vi "Cleanup.vi"(8 "error in (no error)":errorcluster, 11 "DC Brick in":refnum<class "DC Brick.lvclass">) -> (0 "error out":errorcluster)   [LabVIEW 2011, in "Tinkerforge.lvlib" / "DC Brick.lvclass"]
doc: "This VI is the child implementation of \"Cleanup.vi\" and releases all synchronization objects of this child object."
uses:
  DC Brick.lvclass
  DC Brick.lvclass/DC Brick.ctl
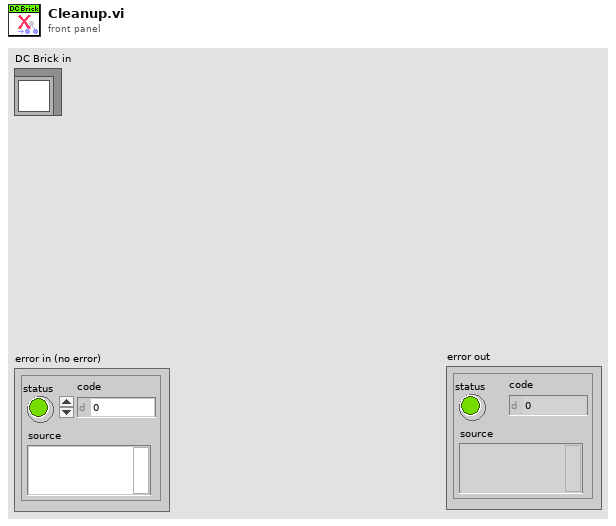
[diagram p1: front panel]
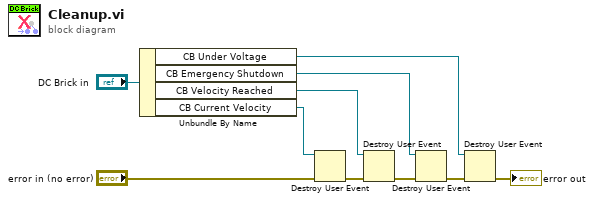
[diagram p0: block diagram]
diagram:
  n1 = Unbundle By Name("DC Brick in") -> ("CB Under Voltage"=w1:refnum<user-event>, "CB Emergency Shutdown"=w2:refnum<user-event>, "CB Velocity Reached"=w6:refnum<user-event>, "CB Current Velocity"=w8:refnum<user-event>)
  n2 = Destroy User Event(user event=w8, error in="error in (no error)") -> (error out=w7:errorcluster)
  n3 = Destroy User Event(user event=w6, error in=w7) -> (error out=w4:errorcluster)
  n4 = Destroy User Event(user event=w2, error in=w4) -> (error out=w5:errorcluster)
  n5 = Destroy User Event(user event=w1, error in=w5) -> (error out=→"error out":errorcluster)
